vi "Move Label to Left.vi"(8 "error in (no error)":errorcluster, 11 "ControlReferenceConstant in":refnum<vi>) -> (0 "error out":errorcluster, 3 "ControlReferenceConstant out":refnum<vi>)   [LabVIEW 2020, in "Add to Private Data.lvlib"]
uses:
  Add to Private Data.lvlib
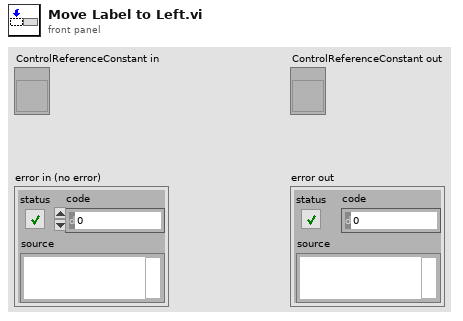
[diagram p1: front panel]
types:
  T1 = typedef "LVPositionTypeDef.ctl" = cluster{"Left":i32, "Top":i32}
  T2 = typedef "LVRectTypeDef.ctl" = cluster{"Left":i16, "Top":i16, "Right":i16, "Bottom":i16}
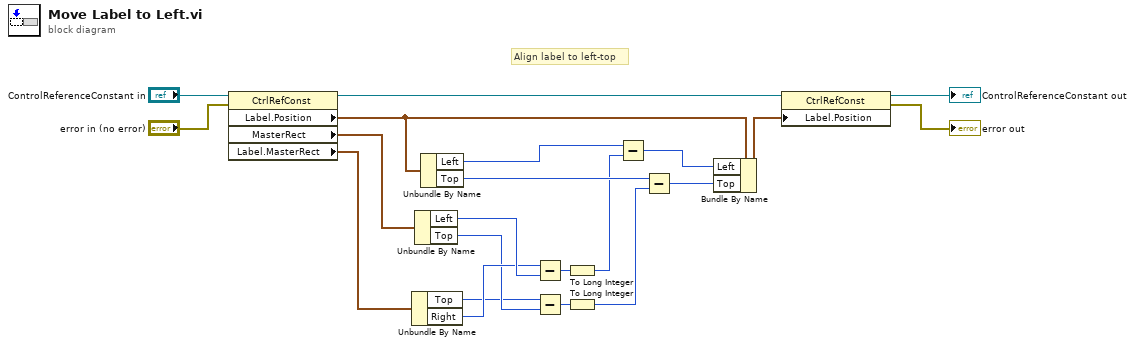
[diagram p0: block diagram]
diagram:
  # "Align label to left-top"
  n1 = property on="Property Node" class="CtrlRefConst"(reference="ControlReferenceConstant in", error in="error in (no error)") -> (reference out=w18:refnum<vi>, "Label.Position"=w1:T1, "MasterRect"=w19:T2, "Label.MasterRect"=w15:T2)  [unwired: 1 out]
  n2 = Unbundle By Name(w15) -> ("Top"=w5:i16, "Right"=w13:i16)
  n3 = Unbundle By Name(w19) -> ("Left"=w14:i16, "Top"=w6:i16)
  n4 = Unbundle By Name(w1) -> ("Left"=w12:i32, "Top"=w7:i32)
  n5 = Subtract(x=w13, y=w14) -> (x-y=w11:i16)
  n6 = Subtract(x=w5, y=w6) -> (x-y=w4:i16)
  n7 = To Long Integer(number=w11) -> (32bit integer=w2:i32)
  n8 = To Long Integer(number=w4) -> (32bit integer=w3:i32)
  n9 = Subtract(x=w12, y=w2) -> (x-y=w10:i32)
  n10 = Subtract(x=w7, y=w3) -> (x-y=w8:i32)
  n11 = Bundle By Name(cluster=w1, "Left"=w10, "Top"=w8) -> (w9:T1)
  n12 = property on="Property Node" class="CtrlRefConst"(reference=w18, "Label.Position"=w9) -> (reference out=→"ControlReferenceConstant out":refnum<vi>, error out=→"error out":errorcluster)  [unwired: 1 in]
